vi "Initialize from Variant.vi"(8 "error in (no error)":errorcluster, 9 "vectors":variant[](array[variant]), 10 "setup data":variant, 11 "Environment.LogFile in":refnum<class "Environment.LogFile.lvclass">) -> (0 "error out":errorcluster, 3 "Environment.LogFile out":refnum<class "Environment.LogFile.lvclass">)   [LabVIEW 2018, in "Environment.LogFile.lvclass"]
uses:
  Environment.LogFile.lvclass
  Environment.LogFile.lvclass/Environment.LogFile.ctl
  <vilib>/addons/_JKI.lib/Serialization/JSON/JKI JSON Serialization.lvlib
panel:
  # "Connector Pane"
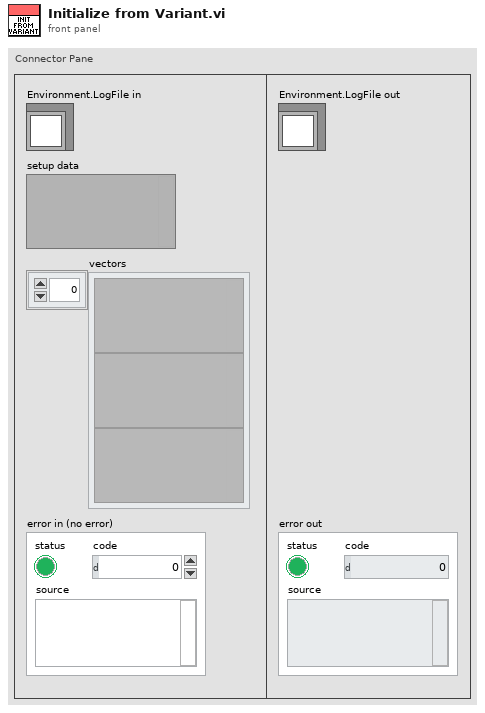
[diagram p1: front panel]
types:
  T1 = typedef "Environment.LogFile.lvclass/Setup Data.ctl" = cluster{"log directory":path, "result directory":path}
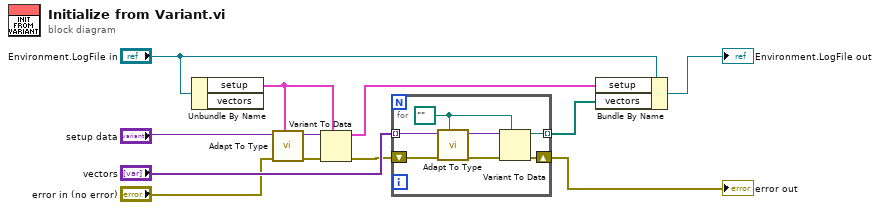
[diagram p0: block diagram]
diagram:
  n1 = Unbundle By Name("Environment.LogFile in") -> ("setup"=w9:T1)  [unwired: 1 out]
  n2 = call <vilib>:"Adapt To Type.vi"("Type and Defaults"=w9, "error in (no error)"="error in (no error)", "Variant in"="setup data") -> ("error out"=w11:errorcluster, "Variant out"=w10:variant)  [unwired: 7 in]
  n3 = Variant To Data(error in=w11, type=w9, Variant=w10) -> (data=w6:T1, error out=w3:errorcluster)
  n4 = for {
    tunnel: [w19] -> w5 mode=indexing
    tunnel: "vectors" -> [w15] mode=indexing
    shift-right: [w17] -> w2
    shift-left: w3 -> [w18]
    w13 = path ""
    n5 = call <vilib>:"Adapt To Type.vi"("Type and Defaults"=w13, "error in (no error)"=w18, "Variant in"=w15) -> ("error out"=w16:errorcluster, "Variant out"=w14:variant)  [unwired: 7 in]
    n6 = Variant To Data(error in=w16, type=w13, Variant=w14) -> (data=w19:path, error out=w17:errorcluster)
  }
  "error out" <- w2
  n7 = Bundle By Name(cluster="Environment.LogFile in", "setup"=w6, "vectors"=w5) -> (→"Environment.LogFile out":refnum<class "Environment.LogFile.lvclass">)
